vi "ALU-FINAL.vi"(5 "Reset Button":bool, 6 "?":bool, 7 "C":bool, 8 "C":T2, 9 "B":T3, 10 "A":T4) -> (0 "Type":bool, 1 "ZF":bool, 2 "CF":bool, 3 "Q":T1, 4 "ERROR":bool)   [LabVIEW 2017]
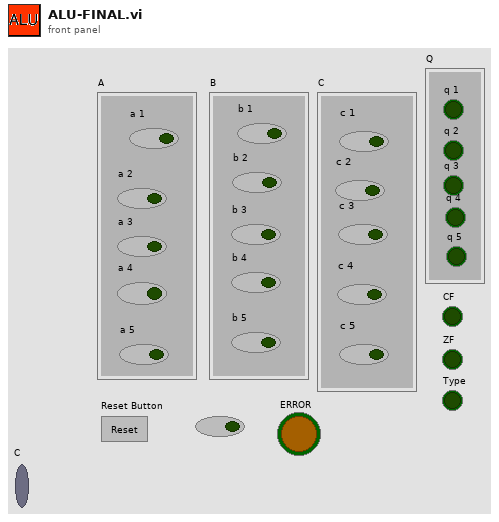
[diagram p1: front panel]
types:
  T1 = cluster{"q 1":bool, "q 2":bool, "q 3":bool, "q 4":bool, "q 5":bool}
  T2 = cluster{"c 1":bool, "c 2":bool, "c 3":bool, "c 4":bool, "c 5":bool}
  T3 = cluster{"b 1":bool, "b 2":bool, "b 3":bool, "b 4":bool, "b 5":bool}
  T4 = cluster{"a 1":bool, "a 2":bool, "a 3":bool, "a 4":bool, "a 5":bool}
  T5 = cluster{"Q 0":bool, "Q 1":bool, "Q 2":bool, "Q 3":bool, "Q 4":bool}
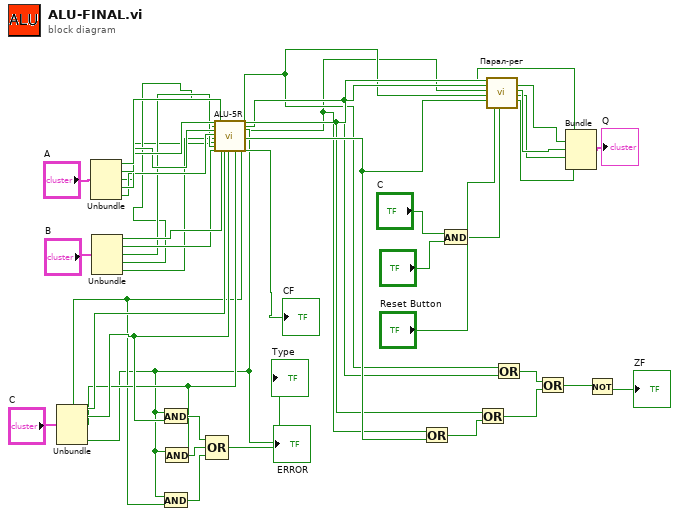
[diagram p0: block diagram]
diagram:
  n1 = Unbundle("C") -> ("c 1"=w10:bool, "c 2"=w9:bool, "c 3"=w8:bool, "c 4"=w7:bool, "c 5"=w6:bool)
  "Type" <- w6
  n2 = Unbundle("A") -> ("a 1"=w19:bool, "a 2"=w18:bool, "a 3"=w2:bool, "a 4"=w17:bool, "a 5"=w16:bool)
  n3 = Unbundle("B") -> ("b 1"=w15:bool, "b 2"=w14:bool, "b 3"=w13:bool, "b 4"=w12:bool, "b 5"=w11:bool)
  n4 = And(x=w6, y=w9) -> (x .and. y?=w32:bool)
  n5 = And(x=w6, y=w7) -> (x .and. y?=w31:bool)
  n6 = And(x=w6, y=w8) -> (x .and. y?=w30:bool)
  n7 = Compound Arithmetic op=OR(w32, w30, w31) -> (→"ERROR":bool)
  n8 = call "ALU-5R.vi"("a  2"=w18, "a  3"=w2, "a  4"=w17, "a  5"=w16, "B 5"=w11, "B 4"=w12, "B 3"=w13, "B 2"=w14, "a 1"=w19, "B 1"=w15, "C 1"=w10, "C 2"=w9, "C 3"=w8, "C 4"=w7, "C 5"=w6) -> ("r 1"=w35:bool, "r 2"=w34:bool, "r 3"=w1:bool, "r 4"=w33:bool, "r 5"=w36:bool, "S 1"=→"CF":bool)  [unwired: 7 in]
  n9 = Or(x=w1, y=w36) -> (x .or. y?=w38:bool)
  n10 = And(x="C", y="?") -> (x .and. y?=w4:bool)
  n11 = Or(x=w35, y=w38) -> (x .or. y?=w39:bool)
  n12 = call "Парал-рег.vi"("d 1"=w35, "d 2"=w34, "d 3"=w1, "d 4"=w33, "d 5"=w36, "Reset"="Reset Button", "C"=w4) -> ("Q 0"=w24:bool, "Q 1"=w23:bool, "Q 2"=w22:bool, "Q 3"=w21:bool, "Q 4"=w20:bool)  [unwired: 8 in]
  n13 = Or(x=w33, y=w34) -> (x .or. y?=w40:bool)
  n14 = Or(x=w40, y=w39) -> (x .or. y?=w42:bool)
  n15 = Bundle("Q 0"=w24, "Q 1"=w23, "Q 2"=w22, "Q 3"=w21, "Q 4"=w20) -> (→"Q":T5)  [unwired: 1 in]
  n16 = Not(x=w42) -> (.not. x?=→"ZF":bool)
